vi "Practica4.3_Registros.vi"() -> ()   [LabVIEW 2022 SP3]
panel:
  out "Némero actual aleatorio":dbl(knob) scale=0.0..10.0
  out "Ultimo valor 11":dbl
  out "Ultimo valor 10":dbl
  out "Ultimo valor 9":dbl
  out "Ultimo valor 8":dbl
  out "Ultimo valor 7":dbl
  out "Ultimo valor 6":dbl
  out "Ultimo valor 5":dbl
  out "Ultimo valor 4":dbl
  out "Ultimo valor 3":dbl
  out "Ultimo valor 2":dbl
  out "Ejecuciones":dbl(knob) scale=0.0..50.0
  out "Ultimo valor 1":dbl
  out "Sí se encontró\nNo se encontró":bool
  in  "Valor selec":dbl
  # "Anahí Montserrat Vázquez Padilla \nPráctica 04: Registros\n07/02/2024"
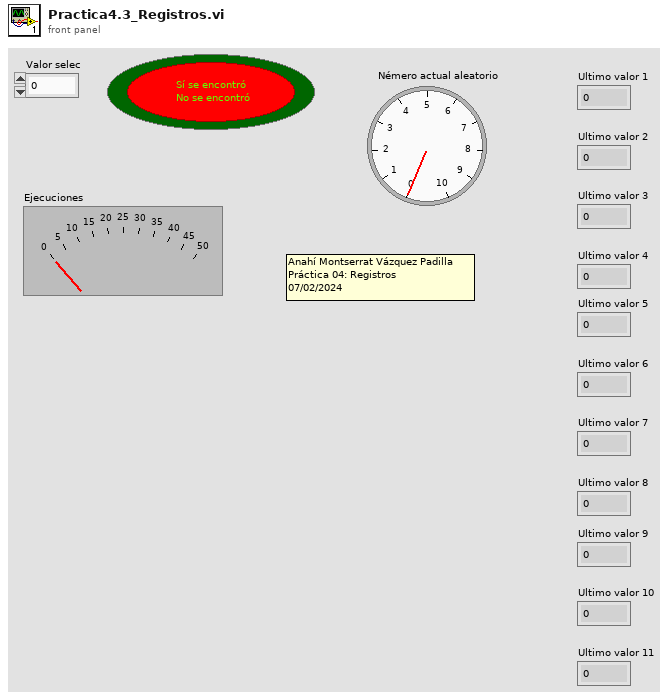
[diagram p1: front panel]
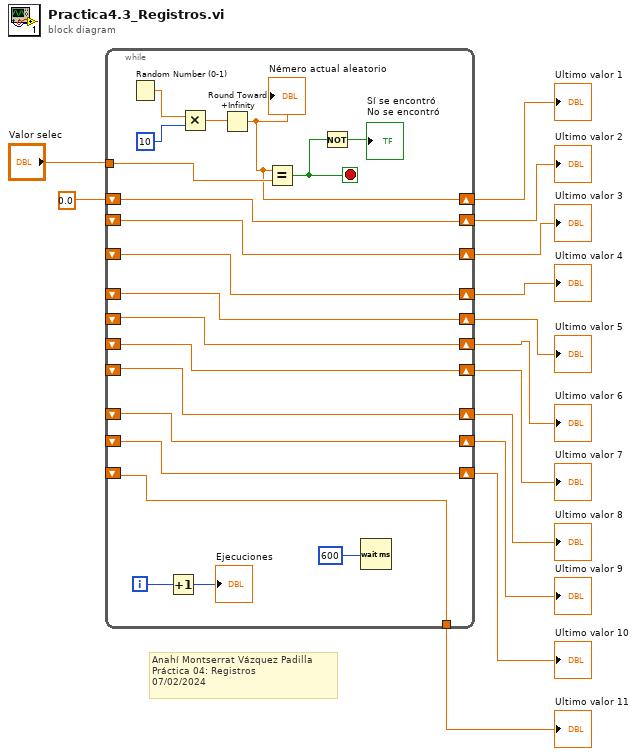
[diagram p0: block diagram]
diagram:
  # "Anahí Montserrat Vázquez Padilla \nPráctica 04: Registros\n07/02/2024"
  n1 = while {
    tunnel: "Valor selec" -> [w30]
    shift-right: [w20] -> w5
    shift-left: _ -> [w19]
    shift-right: [w21] -> w6
    shift-left: _ -> [w20]
    shift-right: [w19] -> w4
    shift-left: _ -> [w18]
    shift-right: [w22] -> w7
    shift-left: _ -> [w21]
    shift-right: [w23] -> w8
    shift-left: _ -> [w22]
    shift-right: [w25] -> w10
    shift-left: _ -> [w24]
    shift-right: [w26] -> w11
    shift-left: _ -> [w25]
    shift-right: [w18] -> w3
    shift-left: _ -> [w17]
    shift-right: [w27] -> w12
    shift-left: 0.0 -> [w26]
    shift-right: [w24] -> w9
    shift-left: _ -> [w23]
    tunnel: [w17] -> w1
    i -> [w29]
    stop <- w15 stop-if-true
    n2 = Random Number (0-1)() -> (number: 0 to 1=w32:dbl)
    n3 = Increment(x=w29) -> (x+1=→"Ejecuciones":i32)
    n4 = Multiply(x=w32, y=10) -> (x*y=w31:dbl)
    n5 = Round Toward +Infinity(x=w31) -> (ceil(x): smallest int >= x=w27:dbl)
    "Némero actual aleatorio" <- w27
    n6 = Equal?(x=w27, y=w30) -> (x = y?=w15:bool)
    n7 = Not(x=w15) -> (.not. x?=→"Sí se encontró\nNo se encontró":bool)
    n8 = Wait (ms)(milliseconds to wait=600) -> ()  [unwired: 1 out]
  }
  "Ultimo valor 1" <- w12
  "Ultimo valor 2" <- w11
  "Ultimo valor 3" <- w10
  "Ultimo valor 4" <- w9
  "Ultimo valor 5" <- w8
  "Ultimo valor 6" <- w7
  "Ultimo valor 7" <- w6
  "Ultimo valor 8" <- w5
  "Ultimo valor 9" <- w4
  "Ultimo valor 10" <- w3
  "Ultimo valor 11" <- w1
